vi "读LabVIEW配置文件.vi"() -> ()   [LabVIEW 2010]
doc: "Illustrates how to read a configuration settings file.\n\nInstructions:\nRun Write Configuration Settings File.vi, located in the file\\config.llb. Then run this VI and select the appropriate configuration settings file to load."
uses:
  <vilib>/Utility/config.llb/Read Key (String).vi
  <vilib>/Utility/config.llb/NI_LVConfig.lvlib
panel:
  out "value":string
  out "found?":bool
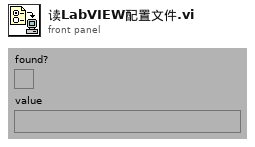
[diagram p1: front panel]
types:
  T1 = typedef "NI_LVConfig.lvlib/Config Data RefNum.ctl" = refnum<k1>
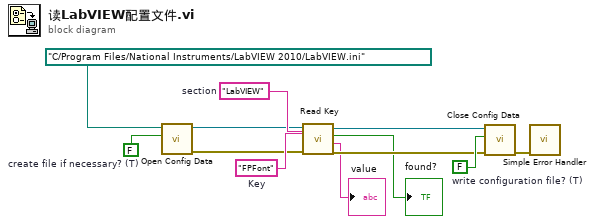
[diagram p0: block diagram]
diagram:
  w7 = "LabVIEW"  # section
  w11 = FALSE  # write configuration file? (T)
  w3 = FALSE  # create file if necessary? (T)
  w6 = "FPFont"  # Key
  n1 = call <vilib>:"Open Config Data.vi"("create file if necessary (T)"=w3, "configuration file path"=path "C:/Program Files/National Instruments/LabVIEW 2010/LabVIEW.ini") -> ("error out"=w2:errorcluster, "refnum"=w1:T1)  [unwired: 7 in, 1 out]
  n2 = call-poly <vilib>:"Read Key.vi"("section"=w7, "error in (no error)"=w2, "key"=w6, "refnum"=w1) -> ("error out"=w10:errorcluster, "value"=→"value":string, "found?"=→"found?":bool, "refnum out"=w9:T1)  [unwired: 4 in]
  n3 = call <vilib>:"Close Config Data.vi"("error in (no error)"=w10, "write file if changed (T)"=w11, "refnum"=w9) -> ("error out"=w12:errorcluster)  [unwired: 7 in, 1 out]
  n4 = call <vilib>:"Simple Error Handler.vi"("error in (no error)"=w12) -> ()  [unwired: 4 in, 5 out]
